vi "PH_SHS_Analysis_Calibrator.calculate Result.vi"(0 "i ref in":refnum<vi>, 5 "error in":errorcluster) -> (14 "i ref out":refnum<vi>, 19 "error out":errorcluster)   [LabVIEW 2014, in "PH_SHS_Analysis_Calibrator.lvlib"]
uses:
  PH_SHS_Analysis_Calibrator.lvlib
  User/Eisenbarth/SHS_v4/SHS_Analysis_Calibrator/SHS_Analysis_Calibrator.lvlib
  User/Eisenbarth/SHS_v4/SHS_Common/SHS_Common.lvlib
  PH_Common/PH_Common.lvlib
  PH_Img_BaseClass/PH_Img_BaseClass.lvlib
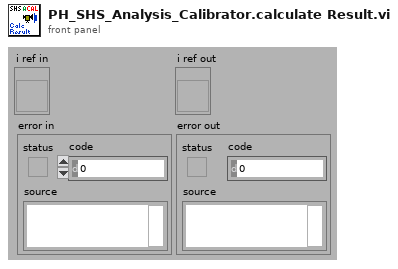
[diagram p1: front panel]
types:
  T1 = typedef "PH_SHS_Analysis_Calibrator.lvlib/PH_SHS_Analysis_Calibrator.i attribute.ctl" = cluster{"GUI Refs":cluster{"Available Cams":refnum<vi>, "OK":refnum<vi>, "Skip":refnum<vi>, "Repeat":refnum<vi>, "Cancel":refnum<vi>, "Dialog":refnum<vi>, "Enough Images?":refnum<vi>}, "Cam instances":string[], "Status":cluster{"#":i32, "Data calculated":bool, "Wanted #":i32}, "IMAQ Image Array":T2[], "Pixel Size [µm]":dbl, "MLA Pitch [µm]":dbl, "Method":enum16{"automatic", "manual"}, "Enough Images?":bool, "SHS Reference Result":T3, "Calculation Error":errorcluster}
  T2 = typedef "IMAQ Image.ctl" = refnum<image>
  T3 = typedef "SHS_Common.lvlib/SHSReference.ctl" = cluster{"Reference":T4[][], "Lens Array Pitch [px]":dbl}
  T4 = typedef "SHS_Common.lvlib/ReferencePoint.ctl" = cluster{"Rect":T5, "Point":T6}
  T5 = typedef "SHS_Common.lvlib/Rectangle.ctl" = cluster{"Left":i32, "Top":i32, "Right":i32, "Bottom":i32}
  T6 = typedef "SHS_Common.lvlib/Point.ctl" = cluster{"x":dbl, "y":dbl, "valid?":bool, "weight":dbl}
  T7 = typedef "PH_Img_BaseClass.lvlib/PH_Img_BaseClass.i attribute.ctl" = cluster{"GUI Refs":T8, "Timeout Image [ms]":i32, "Default Periodic Period [ms]":i32, "Camera":cluster{"Instancename":string, "Notifier":refnum<notifier>}, "Palette":T9, "Cam Settings":cluster{"Cam ID":string, "Gain":dbl, "Brightness":dbl, "Shutter":dbl, "Cam Info Failure":bool, "Mode":i32}}
  T8 = typedef "PH_Img_BaseClass.lvlib/PH_Img_BaseClass.GUI Refs.ctl" = cluster{"Timeout":refnum<vi>, "Image":refnum<vi>, "Palette":refnum<vi>, "Timeout Set":refnum<vi>}
  T9 = typedef "PH_Img_BaseClass.lvlib/PH_Img_BaseClass.Palette.ctl" = i32
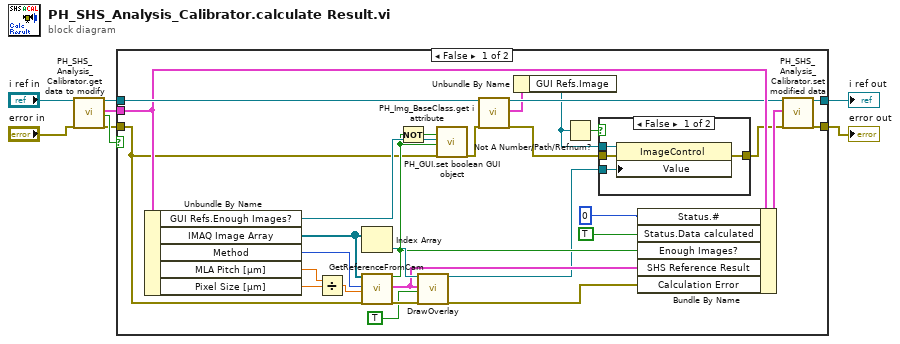
[diagram p0: block diagram]
diagram:
  n1 = call "PH_SHS_Analysis_Calibrator.get data to modify.vi"("i ref in"="i ref in", "error in (no error)"="error in") -> ("i ref out"=w8:refnum<vi>, "i attribute"=w5:T1, "timed out"=w7:bool, "error out"=w6:errorcluster)  [unwired: 14 in]
  n2 = case shown="False" w7 {
    tunnel: w5 -> [w31 _]
    tunnel: w6 -> [w17 w43]
    tunnel: w8 -> [w37 w44]
    tunnel: [w20 w43] -> w2
    tunnel: [w19 w44] -> w1
    frame False {
      n3 = Unbundle By Name(w31) -> ("GUI Refs.Enough Images?"=w24:refnum<vi>, "IMAQ Image Array"=w14:T2[], "Method"=w27:enum16{"automatic", "manual"}, "MLA Pitch [µm]"=w29:dbl, "Pixel Size [µm]"=w30:dbl)
      n4 = Divide(x=w29, y=w30) -> (x/y=w28:dbl)
      n5 = Index Array(array=w14) -> (element=w26:T2)  [unwired: 1 in]
      n6 = call "GetReferenceFromCam.vi"("IMAQ Images"=w14, "Method (auto)"=w27, "MLA Pitch [px]"=w28, "error in (no error)"=w17) -> ("Enough Images?"=w23:bool, "SHS Reference"=w25:T3, "error out"=w33:errorcluster)  [unwired: 13 in]
      n7 = Not(x=w23) -> (.not. x?=w15:bool)
      n8 = call "DrawOverlay.vi"("Image"=w26, "SHS Reference"=w25, "Calibration Mode (false)"=TRUE, "error in (no error)"=w33) -> ("Image Out"=w21:T2, "error out"=w16:errorcluster)  [unwired: 14 in]
      n9 = call "PH_GUI.set boolean GUI object.vi"("Visible (true)"=w15, "Boolean Knob GUI Ref"=w24, "Value"=w23, "error in (no error)"=w17) -> ("error out"=w12:errorcluster)  [unwired: 15 in]
      n10 = call "PH_Img_BaseClass.get i attribute.vi"("i ref in"=w37, "error in (no error)"=w12) -> ("i ref out"=w13:refnum<vi>, "i attribute"=w10:T7, "error out"=w11:errorcluster)  [unwired: 15 in]
      n11 = Unbundle By Name(w10) -> ("GUI Refs.Image"=w9:refnum<vi>)
      n12 = Not A Number/Path/Refnum?(number/path/refnum=w9) -> (NaN/Path/Refnum?=w18:bool)
      n13 = case shown="False" w18 {
        tunnel: w11 -> [w41 w42]
        tunnel: [w40 w42] -> w22
        tunnel: w9 -> [w39 _]
        tunnel: w21 -> [w38 _]
        frame False {
          n14 = property class="ImageControl"(reference=w39, error in=w41, "Value"=w38) -> (error out=w40:errorcluster)  [unwired: 1 out]
        }
        frame True {
        }
      }
      n15 = Bundle By Name(cluster=w31, "Status.#"=0 ("Dark Pics.#"), "Status.Data calculated"=TRUE ("Dark Pics.BI taken"), "Enough Images?"=w23, "SHS Reference Result"=w25, "Calculation Error"=w16) -> (w36:T1)
      n16 = call "PH_SHS_Analysis_Calibrator.set modified data.vi"("i ref in"=w13, "i attribute"=w36, "error in (no error)"=w22) -> ("i ref out"=w19:refnum<vi>, "error out"=w20:errorcluster)  [unwired: 15 in]
    }
    frame True {
    }
  }
  "error out" <- w2
  "i ref out" <- w1
